vi "Cleanup.vi"(8 "error in (no error)":errorcluster, 11 "Start Spot Free Rinse in":refnum<class "Stop Spot Free Rinse.lvclass">) -> (0 "error out":errorcluster, 3 "Start Spot Free Rinse out":refnum<class "Stop Spot Free Rinse.lvclass">)   [LabVIEW 2019, in "Stop Spot Free Rinse.lvclass"]
uses:
  <vilib>/gpm_packages/@cs/Car-wash/Source/Process Steps/Stop Spot Free Rinse/Stop Spot Free Rinse.lvclass
  <vilib>/gpm_packages/@cs/Car-wash/Source/iProcess Step Model/iProcess Step Model/iProcess Step Model.lvclass
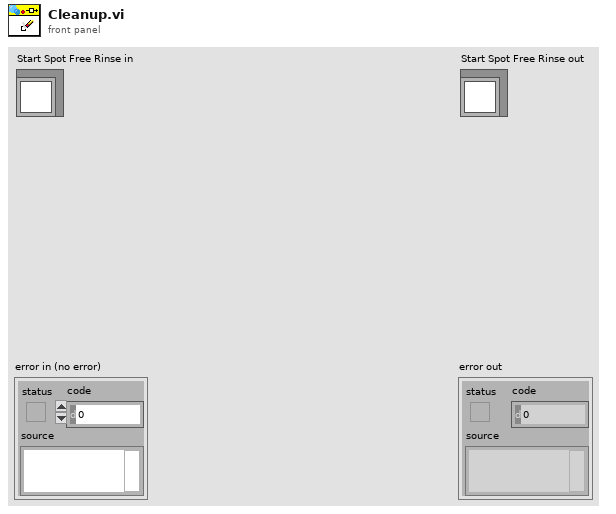
[diagram p1: front panel]
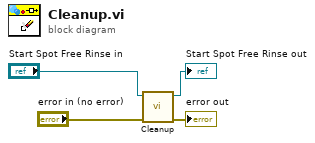
[diagram p0: block diagram]
diagram:
  n1 = call-parent "Cleanup.vi"("error in (no error)"="error in (no error)", "iProcess Step Model in"="Start Spot Free Rinse in") -> ("error out"=→"error out":errorcluster, "iProcess Step Model out"=→"Start Spot Free Rinse out":refnum<class "Stop Spot Free Rinse.lvclass">)  [unwired: 8 in]
